vi "Parse SINGLE.vi"(8 "error in":errorcluster, 10 "read buffer":string) -> (0 "error out":errorcluster, 2 "Measurement":T1)   [LabVIEW 2019, in "AH2500A.lvclass"]
uses:
  AH2500A.lvclass
  Typedefs/AH2500A Measurement--Cluster.ctl
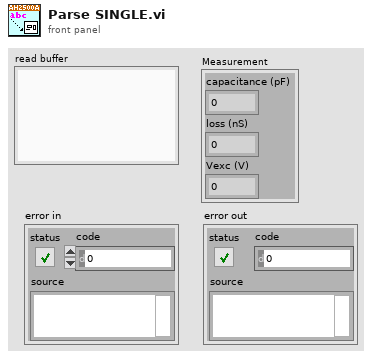
[diagram p1: front panel]
types:
  T1 = typedef "AH2500A.lvclass/AH2500A Measurement--Cluster.ctl" = cluster{"capacitance (pF)":dbl, "loss (nS)":dbl, "Vexc (V)":dbl}
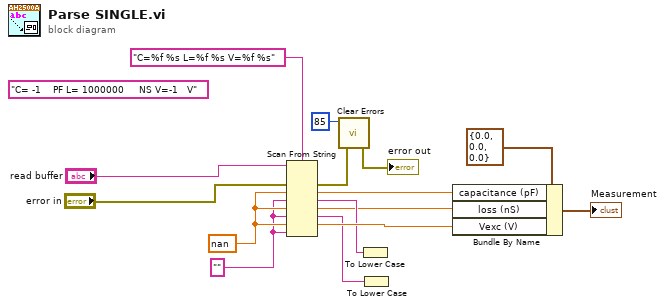
[diagram p0: block diagram]
diagram:
  (unwired) "C= -1    PF L= 1000000     NS V=-1   V" ("t")
  w11 = "" ("default value 2")
  w12 = nan ("default (0 dbl)")
  n1 = Scan From String(format string="C=%f %s L=%f %s V=%f %s", input string="read buffer", error in="error in", default 1=w12, default 2=w11, default 3=w12, default 4=w11, default 5=w12, default 6=w11) -> (error out=w4:errorcluster, output 1=w10:dbl, output 2=w7:string, output 3=w6:dbl, output 4=w8:string, output 5=w9:dbl)  [unwired: 2 in, 2 out]
  n2 = call <vilib>:"Clear Errors.vi"("error in (no error)"=w4, "specific error code to clear (0: all)"=85) -> ("error out"=→"error out":errorcluster)  [unwired: 4 in, 1 out]
  n3 = To Lower Case(string=w7) -> ()  [unwired: 1 out]
  n4 = To Lower Case(string=w8) -> ()  [unwired: 1 out]
  n5 = Bundle By Name(cluster=T1 {"capacitance (pF)"=0.0, "loss (nS)"=0.0, "Vexc (V)"=0.0} ("Measurement"), "capacitance (pF)"=w10, "loss (nS)"=w6, "Vexc (V)"=w9) -> (→"Measurement":T1)
